vi "4-temp2.vi"(3 "this":i32, 4 "button":i32, 5 "shift in":bool) -> (0 "next state":i32, 1 "shift out":bool)   [LabVIEW 2017]
panel:
  out "setting out":T1
  in  "setting in":T1={"Auto1"=TRUE, "Auto2"=TRUE, "Rel1"=TRUE, "Rel2"=TRUE, "Filt1"=TRUE, "Filt2"=TRUE, "Rate"=enum."Slow", "Range1"=enum."10mV", "Range2"=enum."100mV", "Filt3"=TRUE, "Filt4"=TRUE, "Rel temp 1"=TRUE, "Analog1"=FALSE, "Analog2"=FALSE, "Analog temp 1"=FALSE, "Digital1"=TRUE, "Digital2"=TRUE, "Digital temp 1 "=TRUE, "Window1"=enum."0,01%", "Window2"=enum."0,01%", "Window temp 1"=enum."0,01%", "RDGS1"="010", "RDGS2"="010", "RDGS temp 1"="010", "Type_type1"=TRUE, "Type_type2"=TRUE, "Type_type temp 1"=TRUE, "LSync"=FALSE, "Unit"=enum."C", "Sens"=TRUE, "Type tcoupl"=enum."J", "Junc"=TRUE, "prevState"=0, "Rel temp 2"=TRUE, "Analog temp 2"=FALSE, "Digital temp 2"=TRUE, "Type_type temp 2"=TRUE, "RDGS temp 2"="010", "Window temp 2"=enum."0,01%", "addres"=0}
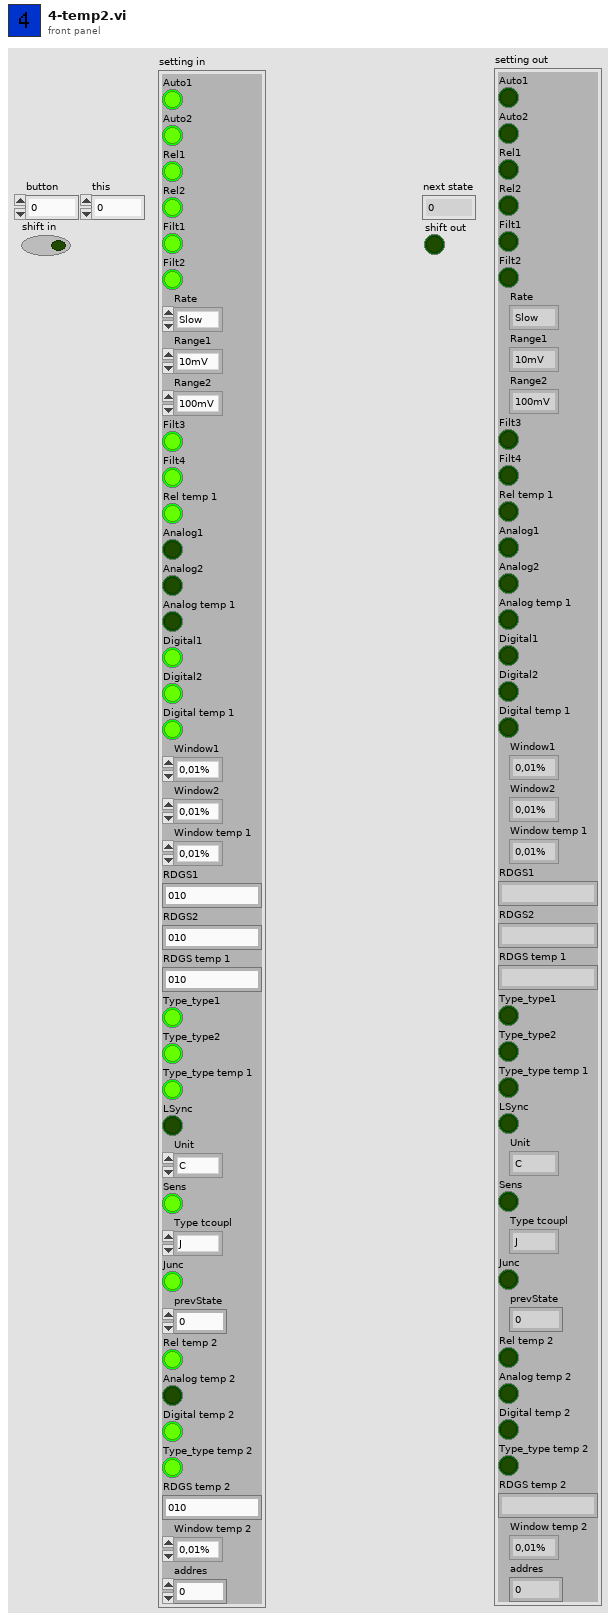
[diagram p1: front panel]
types:
  T1 = cluster{"Auto1":bool, "Auto2":bool, "Rel1":bool, "Rel2":bool, "Filt1":bool, "Filt2":bool, "Rate":enum16{"Slow", "Med", "Fast"}, "Range1":enum16{"10mV", "100mV", "1V", "10V", "100V"}, "Range2":enum16{"100mV", "1V", "10V"}, "Filt3":bool, "Filt4":bool, "Rel temp 1":bool, "Analog1":bool, "Analog2":bool, "Analog temp 1":bool, "Digital1":bool, "Digital2":bool, "Digital temp 1 ":bool, "Window1":enum16{"0,01%", "0,1%", "1%", "10%", "None"}, "Window2":enum16{"0,01%", "0,1%", "1%", "10%", "None"}, "Window temp 1":enum16{"0,01%", "0,1%", "1%", "10%", "None"}, "RDGS1":string, "RDGS2":string, "RDGS temp 1":string, "Type_type1":bool, "Type_type2":bool, "Type_type temp 1":bool, "LSync":bool, "Unit":enum16{"C", "K", "F"}, "Sens":bool, "Type tcoupl":enum16{"J", "K", "T", "E", "R", "S", "B", "N"}, "Junc":bool, "prevState":i32, "Rel temp 2":bool, "Analog temp 2":bool, "Digital temp 2":bool, "Type_type temp 2":bool, "RDGS temp 2":string, "Window temp 2":enum16{"0,01%", "0,1%", "1%", "10%", "None"}, "addres":i32}
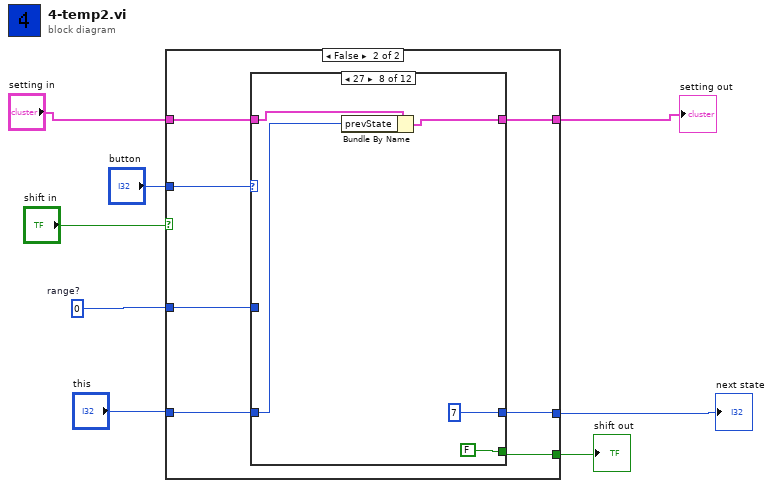
[diagram p0: block diagram]
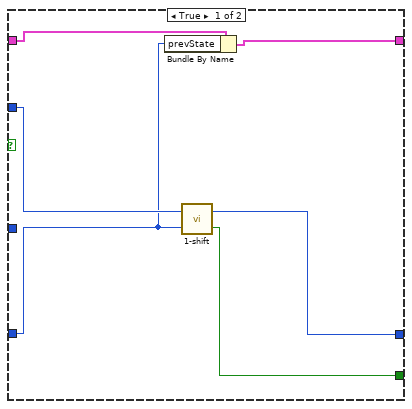
[diagram p2: hidden frame]
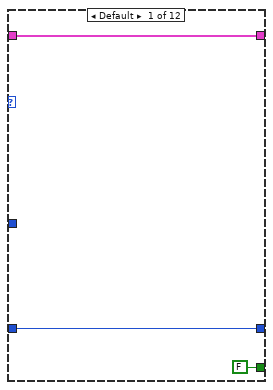
[diagram p3: hidden frame]
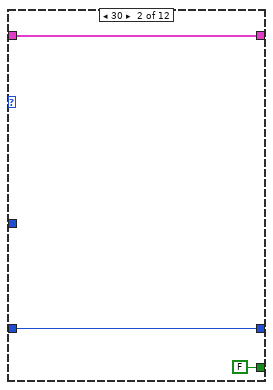
[diagram p4: hidden frame]
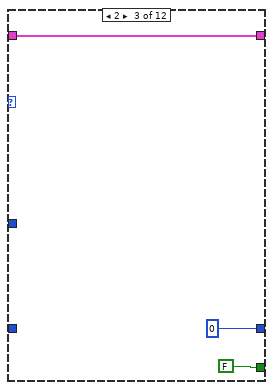
[diagram p5: hidden frame]
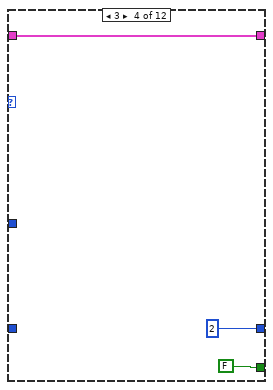
[diagram p6: hidden frame]
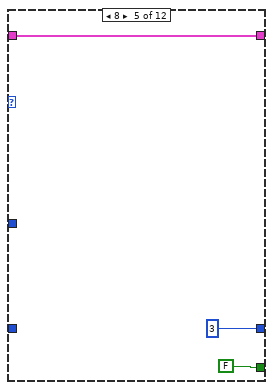
[diagram p7: hidden frame]
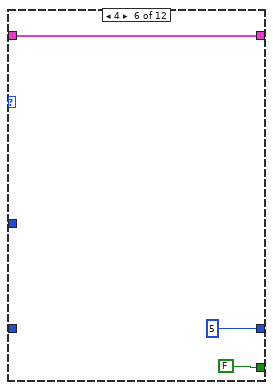
[diagram p8: hidden frame]
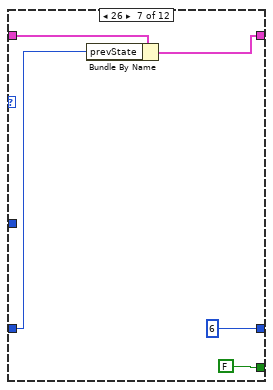
[diagram p9: hidden frame]
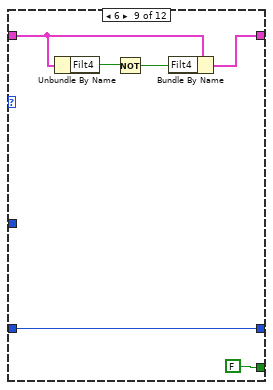
[diagram p10: hidden frame]
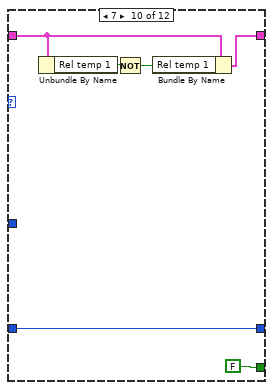
[diagram p11: hidden frame]
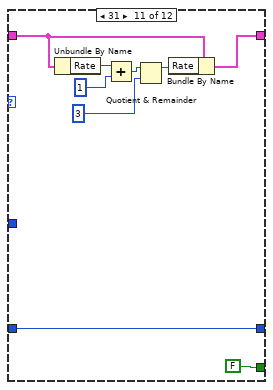
[diagram p12: hidden frame]
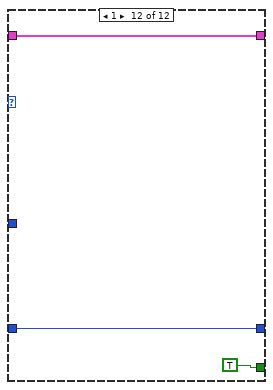
[diagram p13: hidden frame]
diagram:
  w3 = 0  # range?
  n1 = case shown="False" "shift in" {
    tunnel: "button" -> [w14 w21]
    tunnel: [w13 w20] -> w6
    tunnel: "this" -> [w9 w19]
    tunnel: [w12 w18] -> w4
    tunnel: "setting in" -> [w11 w17]
    tunnel: [w10 w16] -> w2
    tunnel: w3 -> [_ w15]
    frame True {
      n2 = Bundle By Name(cluster=w11, "prevState"=w9) -> (w10:T1)
      n3 = call "1-shift.vi"("this"=w9, "button"=w14) -> ("shift"=w12:bool, "next state"=w13:i32)
    }
    frame False {
      n4 = case shown="27" w21 {
        tunnel: [w23 w26 0 2 3 5 6 7 w54 w60 w69 w73] -> w20
        tunnel: w19 -> [w23 w26 _ _ _ _ w40 w46 w54 w60 w69 w73]
        tunnel: [FALSE ("shift") FALSE ("shift") FALSE ("shift") FALSE ("shift") FALSE ("shift") FALSE ("shift") FALSE ("shift") FALSE ("shift") FALSE ("shift") FALSE ("shift") FALSE ("shift") TRUE ("shift")] -> w18
        tunnel: w17 -> [w24 w27 w28 w31 w34 w37 w42 w47 w51 w57 w68 w71]
        tunnel: [w24 w27 w28 w31 w34 w37 w41 w45 w50 w56 w67 w71] -> w16
        tunnel: w15 -> [_ _ _ _ _ _ _ _ _ _ _ _]
        frame Default {
        }
        frame 30 {
        }
        frame 2 {
        }
        frame 3 {
        }
        frame 8 {
        }
        frame 4 {
        }
        frame 26 {
          n5 = Bundle By Name(cluster=w42, "prevState"=w40) -> (w41:T1)
        }
        frame 27 {
          n6 = Bundle By Name(cluster=w47, "prevState"=w46) -> (w45:T1)
        }
        frame 6 {
          n7 = Unbundle By Name(w51) -> ("Filt4"=w53:bool)
          n8 = Not(x=w53) -> (.not. x?=w52:bool)
          n9 = Bundle By Name(cluster=w51, "Filt4"=w52) -> (w50:T1)
        }
        frame 7 {
          n10 = Unbundle By Name(w57) -> ("Rel temp 1"=w59:bool)
          n11 = Not(x=w59) -> (.not. x?=w58:bool)
          n12 = Bundle By Name(cluster=w57, "Rel temp 1"=w58) -> (w56:T1)
        }
        frame 31 {
          n13 = Unbundle By Name(w68) -> ("Rate"=w66:enum16{"Slow", "Med", "Fast"})
          n14 = Add(x=w66, y=1) -> (x+y=w64:i32)
          n15 = Quotient & Remainder(x=w64, y=3) -> (x-y*floor(x/y)=w63:i32)  [unwired: 1 out]
          n16 = Bundle By Name(cluster=w68, "Rate"=w63) -> (w67:T1)
        }
        frame 1 {
        }
      }
    }
  }
  "next state" <- w6
  "shift out" <- w4
  "setting out" <- w2
